vi "ProjectClose.vi"(8 "error in (no error)":errorcluster, 11 "Project Ref in":T1) -> (0 "error out":errorcluster)   [LabVIEW 2015, in "MiscHelperVIs.lvlib"]
uses:
  MiscHelperVIs.lvlib
  <vilib>/NI Veristand/Execution/Project/Project Ref.ctl
  NationalInstruments.VeriStand.ClientAPI
  <vilib>/NI Veristand/Execution/Project/NI_VS Project ExecutionAPI.lvlib
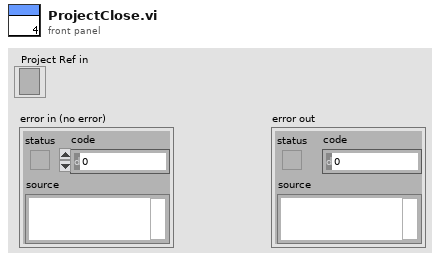
[diagram p1: front panel]
types:
  T1 = typedef "NI_VS Project ExecutionAPI.lvlib/Project Ref.ctl" = refnum<k24>
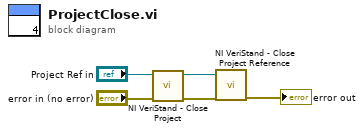
[diagram p0: block diagram]
diagram:
  n1 = call <vilib>:"NI VeriStand - Close Project.vi"("error in (no error)"="error in (no error)", "Project Ref in"="Project Ref in") -> ("error out"=w4:errorcluster, "Project Ref out"=w5:T1)  [unwired: 8 in]
  n2 = call <vilib>:"NI VeriStand - Close Project Reference.vi"("error in (no error)"=w4, "Project Ref"=w5) -> ("error out"=→"error out":errorcluster)  [unwired: 9 in]
